vi "Climb_Motors.vi"(8 "Right Bottom Right":bool, 9 "Right Bottom Left":bool, 10 "Right Top Left":bool, 11 "Right Top Right":bool) -> ()   [LabVIEW 2020]
uses:
  <vilib>/Rock Robotics/WPI/ThirdParty/Phoenix-LabVIEW/Motor Controller/Controls/CTRE_Phoenix_MotorControl_ControlMode.ctl
  <vilib>/Rock Robotics/WPI/ThirdParty/Phoenix-LabVIEW/Motor Controller/Get/CTRE_Phoenix_MotorController_IntegratedSensorData_TalonFX.vi
  <vilib>/addons/control/pid/pid.llb/PID (DBL).vi
  <vilib>/addons/control/pid/NI_PID_pid.lvlib
panel:
  in  "Inches 2":dbl=27.5
  in  "PID gains 2":T1={"proportional gain (Kc)"=3e-05, "integral time (Ti, min)"=0.0, "derivative time (Td, min)"=2e-05} {"derivative time (Td, min)" format="%.6f"; "integral time (Ti, min)" format="%.3f"; "proportional gain (Kc)" format="%.7f"}
  in  "PID gains":T1={"proportional gain (Kc)"=3e-05, "integral time (Ti, min)"=0.0, "derivative time (Td, min)"=2e-05} {"derivative time (Td, min)" format="%.6f"; "integral time (Ti, min)" format="%.3f"; "proportional gain (Kc)" format="%.7f"}
  in  "Inches":dbl=27.5
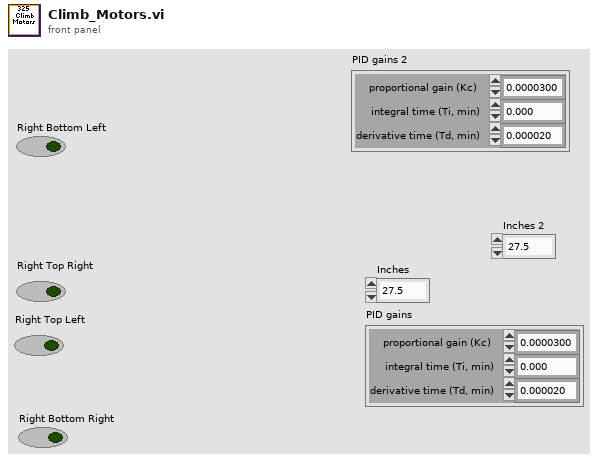
[diagram p1: front panel]
types:
  T1 = cluster{"proportional gain (Kc)":dbl, "integral time (Ti, min)":dbl, "derivative time (Td, min)":dbl}
  T2 = enum16{"FollowerType_PercentOutput", "FollowerType_AuxOutput1"}
  T3 = typedef "CTRE_Phoenix_MotorControl_ControlMode.ctl" = u16
  T4 = typedef "WPI_MotorControlDeviceRef.ctl" = cluster{"DeviceStatus":errorcluster, "Type":T5, "PWM":cluster{"PWM Channel":T6, "DeadBand":T7}, "CAN":cluster{"Device Number":u8, "SetOutput VI Ref":variant, "GetOutput VI Ref":variant, "Enable VI Ref":variant, "Disable VI Ref":variant, "Data":variant}, "Invert":bool, "DIO PWM":cluster{"PWM \"Enable\" Channel":T6, "DIOChannel":T8, "PWM Rate":dbl}}
  T5 = typedef "WPI_MotorControlType.ctl" = enum16{"PWM", "CAN", "DIO PWM"}
  T6 = typedef "FPGA_DIOPWMChannel.ctl" = enum8{"PWM 0", "PWM 1", "PWM 2", "PWM 3", "PWM 4", "PWM 5", "PWM 6", "PWM 7", "PWM 8", "PWM 9", "PWM MXP 0", "PWM MXP 1", "PWM MXP 2", "PWM MXP 3", "PWM MXP 4", "PWM MXP 5", "PWM MXP 6", "PWM MXP 7", "PWM MXP 8", "PWM MXP 9", "Invalid"}
  T7 = typedef "WPI_PWMDeadband.ctl" = cluster{"Name":string, "maxPositivePwm":i32, "minPositivePwm":i32, "centerPwm":i32, "maxNegativePwm":i32, "minNegativePwm":i32, "angularRange":u16}
  T8 = typedef "FPGA_DIOChannel.ctl" = enum8{"DIO 0", "DIO 1", "DIO 2", "DIO 3", "DIO 4", "DIO 5", "DIO 6", "DIO 7", "DIO 8", "DIO 9", "DIO MXP 0", "DIO MXP 1", "DIO MXP 2", "DIO MXP 3", "DIO MXP 4", "DIO MXP 5", "DIO MXP 6", "DIO MXP 7", "DIO MXP 8", "DIO MXP 9", "DIO MXP 10", "DIO MXP 11", "DIO MXP 12", "DIO MXP 13", "DIO MXP 14", "DIO MXP 15", "SPI Port CS1", "SPI Port CS2", "SPI Port CS3", "SPI Port MISO", "SPI Port MOSI", "Invalid"}
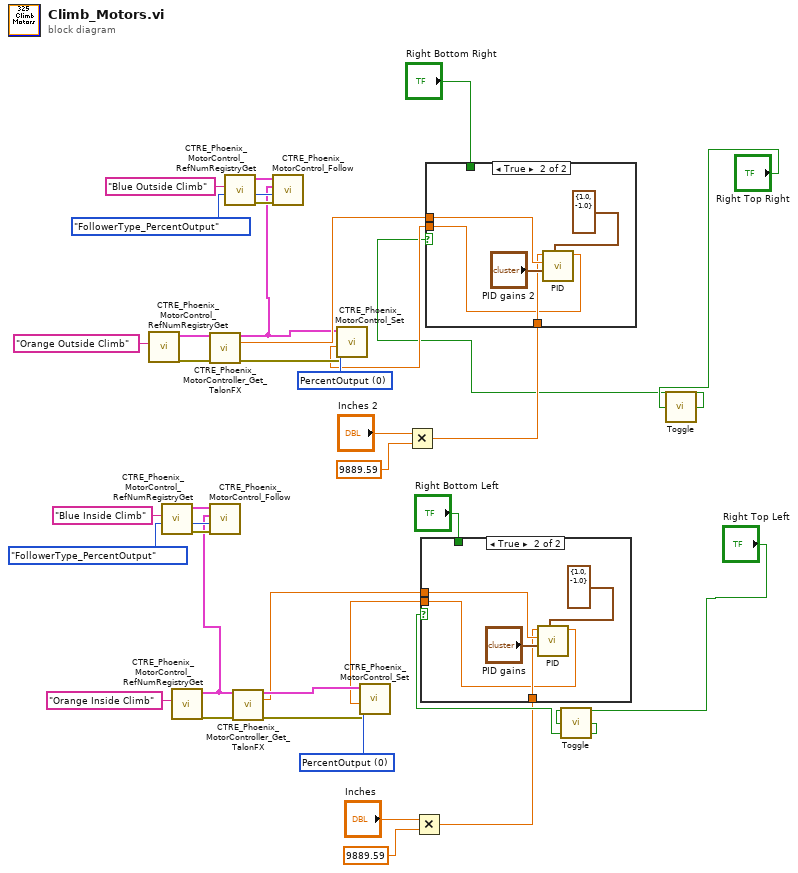
[diagram p0: block diagram]
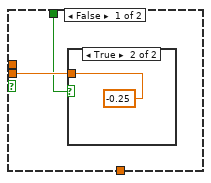
[diagram p2: hidden frame]
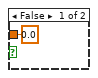
[diagram p3: hidden frame]
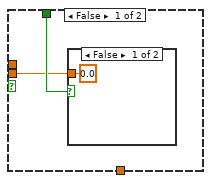
[diagram p4: hidden frame]
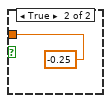
[diagram p5: hidden frame]
diagram:
  w30 = T3 0 items=["PercentOutput"=0, "Position"=1, "Velocity"=2, "Current"=3, "Follower"=5, "MotionProfile"=6, "MotionMagic"=7, "MotionProfileArc"=10, "Disabled"=15] ("Control Mode")
  w35 = T3 0 items=["PercentOutput"=0, "Position"=1, "Velocity"=2, "Current"=3, "Follower"=5, "MotionProfile"=6, "MotionMagic"=7, "MotionProfileArc"=10, "Disabled"=15] ("Control Mode")
  n1 = call <vilib>:"CTRE_Phoenix_MotorControl_RefNumRegistryGet.vi"("refnum name"="Orange Outside Climb") -> ("error out"=w29:errorcluster, "PhoenixMotorControlDevRef"=w11:T4)  [unwired: 9 in]
  n2 = call <vilib>:"CTRE_Phoenix_MotorControl_RefNumRegistryGet.vi"("refnum name"="Blue Inside Climb") -> ("error out"=w5:errorcluster, "PhoenixMotorControlDevRef"=w4:T4)  [unwired: 9 in]
  n3 = call <vilib>:"CTRE_Phoenix_MotorControl_RefNumRegistryGet.vi"("refnum name"="Orange Inside Climb") -> ("error out"=w34:errorcluster, "PhoenixMotorControlDevRef"=w1:T4)  [unwired: 9 in]
  n4 = call-poly <vilib>:"CTRE_Phoenix_MotorController_Get_TalonFX.vi"("PhoenixMotorControlDevRef"=w11, "error in"=w29) -> ("PhoenixMotorControlDevRef"=w2:T4, "Position"=w18:dbl, "error out"=w28:errorcluster)  [unwired: 9 in, 2 out]
  n5 = call <vilib>:"CTRE_Phoenix_MotorControl_Follow.vi"("error in (no error)"=w5, "FollowerType"=T2."FollowerType_PercentOutput", "Master Controller to Follow"=w1, "PhoenixMotorControlDevRef"=w4) -> ()  [unwired: 6 in, 2 out]
  n6 = call <vilib>:"CTRE_Phoenix_MotorControl_RefNumRegistryGet.vi"("refnum name"="Blue Outside Climb") -> ("error out"=w9:errorcluster, "PhoenixMotorControlDevRef"=w8:T4)  [unwired: 9 in]
  n7 = call-poly <vilib>:"CTRE_Phoenix_MotorController_Get_TalonFX.vi"("PhoenixMotorControlDevRef"=w1, "error in"=w34) -> ("PhoenixMotorControlDevRef"=w33:T4, "Position"=w20:dbl, "error out"=w32:errorcluster)  [unwired: 9 in, 2 out]
  n8 = call <vilib>:"CTRE_Phoenix_MotorControl_Follow.vi"("error in (no error)"=w9, "FollowerType"=T2."FollowerType_PercentOutput", "Master Controller to Follow"=w2, "PhoenixMotorControlDevRef"=w8) -> ()  [unwired: 6 in, 2 out]
  n9 = Multiply(x="Inches 2", y=9889.59) -> (x*y=w15:dbl)
  n10 = Multiply(x="Inches", y=9889.59) -> (x*y=w19:dbl)
  n11 = call "Toggle.vi"("Boolean"="Right Top Left") -> ("Boolean Out"=w21:bool)
  n12 = case shown="True" w21 {
    tunnel: [w37 w41] -> w23
    tunnel: "Right Bottom Left" -> [w38 _]
    tunnel: w20 -> [_ w44]
    tunnel: w19 -> [_ w43]
    frame False {
      n13 = case shown="False" w38 {
        tunnel: [0.0 ("output") -0.25 ("output")] -> w37
        frame False {
        }
        frame True {
        }
      }
    }
    frame True {
      n14 = call-poly <vilib>:"PID.vi"("output range"=cluster{"output high":dbl, "output low":dbl} {"output high"=1.0, "output low"=-1.0}, "PID gains"="PID gains", "process variable"=w44, "setpoint"=w43) -> ("output"=w41:dbl)  [unwired: 6 in, 1 out]
    }
  }
  n15 = call <vilib>:"CTRE_Phoenix_MotorControl_Set.vi"("error in (no error)"=w32, "Output"=w23, "Control Mode"=w35, "PhoenixMotorControlDevRef"=w33) -> ()  [unwired: 6 in, 2 out]
  n16 = call "Toggle.vi"("Boolean"="Right Top Right") -> ("Boolean Out"=w13:bool)
  n17 = case shown="True" w13 {
    tunnel: [w47 w50] -> w14
    tunnel: w18 -> [_ w53]
    tunnel: w15 -> [_ w52]
    tunnel: "Right Bottom Right" -> [w46 _]
    frame False {
      n18 = case shown="True" w46 {
        tunnel: [0.0 ("output") -0.25 ("output")] -> w47
        frame False {
        }
        frame True {
        }
      }
    }
    frame True {
      n19 = call-poly <vilib>:"PID.vi"("output range"=cluster{"output high":dbl, "output low":dbl} {"output high"=1.0, "output low"=-1.0}, "PID gains"="PID gains 2", "process variable"=w53, "setpoint"=w52) -> ("output"=w50:dbl)  [unwired: 6 in, 1 out]
    }
  }
  n20 = call <vilib>:"CTRE_Phoenix_MotorControl_Set.vi"("error in (no error)"=w28, "Output"=w14, "Control Mode"=w30, "PhoenixMotorControlDevRef"=w2) -> ()  [unwired: 6 in, 2 out]
